vi "ConvertErrorCodeToErrorName.vi"(11 "ErrorCode":i32) -> (2 "not found":bool, 3 "ErrorName":string)   [LabVIEW 2017]
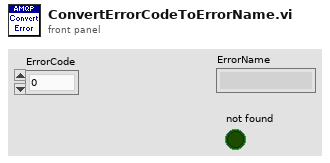
[diagram p1: front panel]
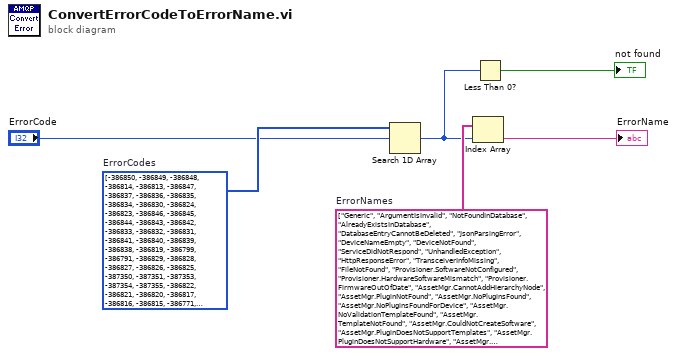
[diagram p0: block diagram]
diagram:
  w6 = i32[] [-386850, -386849, -386848, -386814, -386813, -386847, -386837, -386836, -386835, -386834, -386830, -386824, -386823, -386846, -386845, -386844, -386843, -386842, -386833, -386832, -386831, -386841, -386840, -386839, -386838, -386819, -386799, -386791, -386829, -386828, -386827, -386826, -386825, -387350, -387351, -387353, -387354, -387355, -386822, -386821, -386820, -386817, -386816, -386815, -386771, -386818, -386809, -386810, -386812, -386811, -386808, -386807, -386797, -386796, -386795, -386794, -386806, -386805, -386804, -386803, -386798, -386802, -386801, -386800, -386793, -386792, -386773, -386772, -386790, -386789, -386788, -386787, -386786, -386785, -386784, -386783, -386782, -386781, -386780, -386779, -386778, -386777, -386776, -386775, -386774]  # ErrorCodes
  w4 = string[] ["Generic", "ArgumentIsInvalid", "NotFoundInDatabase", "AlreadyExistsInDatabase", "DatabaseEntryCannotBeDeleted", "JsonParsingError", "DeviceNameEmpty", "DeviceNotFound", "ServiceDidNotRespond", "UnhandledException", "HttpResponseError", "TransceiverInfoMissing", "FileNotFound", "Provisioner.SoftwareNotConfigured", "Provisioner.HardwareSoftwareMismatch", "Provisioner.FirmwareOutOfDate", "AssetMgr.CannotAddHierarchyNode", "AssetMgr.PluginNotFound", "AssetMgr.NoPluginsFound", "AssetMgr.NoPluginsFoundForDevice", "AssetMgr.NoValidationTemplateFound", "AssetMgr.TemplateNotFound", "AssetMgr.CouldNotCreateSoftware", "AssetMgr.PluginDoesNotSupportTemplates", "AssetMgr.PluginDoesNotSupportHardware", "AssetMgr.HierarchyRootNodeAlreadyExists", "AssetMgr.StaleSoftwareVersion", "AssetMgr.ValidationErrors", "Device.WebServiceGetConnectionInfo", "Device.WebServiceSetConnectionInfo", "Device.WebServiceGetHardwareInfo", "Device.WebServiceGetHostname", "Device.WebServiceReboot", "Device.TransCommFileTransferAlreadyInProgress", "Device.TransCommSendFileTimeout", "Device.TransCommFileNotFound", "Device.TransCommNotAuthorized", "Device.TransCommInvalidRefNum", "Auth.VerificationFailure", "Auth.SrpInitiationRequestNotFound", "Auth.EncryptionKeyNotFound", "Auth.RoleNameAlreadyExists", "Auth.RoleNotFound", "Auth.RoleCannotBeDeleted", "Auth.LdapConfigurationNotSet", "Stream.Invalid", "Historian.COMException", "Historian.UnauthorizedAccess", "Historian.PiTagDoesNotExist", "Historian.UnableToCreatePiTag", "Historian.TagPathAlreadyExists", "Historian.PiTagNameAlreadyExists", "Historian.PiTagPatternAlreadyExists", "Historian.PiTagPatternDoesNotExist", "Historian.PiCustomNameObjectIsInvalid", "Historian.UnableToApplyTagPattern", "Storage.DuplicatePacket", "Storage.MissingPacket", "Storage.IOError", "Config.SectionNotFound", "Config.KeyNotFound", "Alarm.RuleNotFound", "Alarm.UserUpdatesNotAllowed", "Deploy.SMSError", "Smtp.TemplateNotFound", "Smtp.AddressGroupNotFound", "Smtp.ToAddressRequired", "Smtp.InvalidServiceConfiguration", "Analysis.StreamPrepError", "Analysis.NotStreamingBlockReceived", "Analysis.NotStreamingStreamStopReceived", "Analysis.UnpackJsonStateStringError", "Analysis.UnknownJsonStateStringMessageType", "Analysis.JsonStateMessageConversionError", "Analysis.FileOpenFailure", "Analysis.HierarchyPropsNotFound", "Analysis.ReferenceChannelNotFound", "Analysis.ReferenceTypeNotFound", "Analysis.SpeedPropertyNotFound", "Analysis.UnknownFeatureCodeName", "Analysis.UnitStringNotFound", "Analysis.UnitConversionUnsuccessful", "Analysis.InvalidAmplitudeScale", "Analysis.SpectralBandCacheError", "Analysis.UnknownInternalMessage"]  # ErrorNames
  n1 = Search 1D Array(1D array=w6, element="ErrorCode") -> (index of element=w2:i32)  [unwired: 1 in]
  n2 = Index Array(array=w4, index=w2) -> (element=→"ErrorName":string)
  n3 = Less Than 0?(x=w2) -> (x < 0?=→"not found":bool)
